vi "check out and in tracking spot.vi"(0 "N spot tracker in":T1, 1 "set state?":bool, 5 "tracking state in":T2={"x state"={"pos estimate"=0.0, "v estimate"=0.0, "weighted position error sum"=0.0, "photon count"=0, "transmit tick count"=0, "axis number"=0, "px (levels^2)"=0.0, "pxv (levels^2/ticks)"=0.0, "pv (levels^2/ticks^2)"=0.0, "vel diff (levels^2/ticks^3)"=0.0, "gx"=0.0, "rtwiddle"=0.0, "photon count ch0"=0, "photon count ch1"=0, "Dx - for pos only k-f"=0.0}, "y state"={"pos estimate"=0.0, "v estimate"=0.0, "weighted position error sum"=0.0, "photon count"=0, "transmit tick count"=0, "axis number"=1, "px (levels^2)"=0.0, "pxv (levels^2/ticks)"=0.0, "pv (levels^2/ticks^2)"=0.0, "vel diff (levels^2/ticks^3)"=0.0, "gx"=0.0, "rtwiddle"=0.0, "photon count ch0"=0, "photon count ch1"=0, "Dx - for pos only k-f"=0.0}, "z state"={"pos estimate"=0.0, "v estimate"=0.0, "weighted position error sum"=0.0, "photon count"=0, "transmit tick count"=0, "axis number"=2, "px (levels^2)"=0.0, "pxv (levels^2/ticks)"=0.0, "pv (levels^2/ticks^2)"=0.0, "vel diff (levels^2/ticks^3)"=0.0, "gx"=0.0, "rtwiddle"=0.0, "photon count ch0"=0, "photon count ch1"=0, "Dx - for pos only k-f"=0.0}}, 7 "new circle":bool, 9 "permission to swap states":bool, 11 "set state value":T2={"x state"={"pos estimate"=0.0, "v estimate"=0.0, "weighted position error sum"=0.0, "photon count"=0, "transmit tick count"=0, "axis number"=0, "px (levels^2)"=0.0, "pxv (levels^2/ticks)"=0.0, "pv (levels^2/ticks^2)"=0.0, "vel diff (levels^2/ticks^3)"=0.0, "gx"=0.0, "rtwiddle"=0.0, "photon count ch0"=0, "photon count ch1"=0, "Dx - for pos only k-f"=0.0}, "y state"={"pos estimate"=0.0, "v estimate"=0.0, "weighted position error sum"=0.0, "photon count"=0, "transmit tick count"=0, "axis number"=1, "px (levels^2)"=0.0, "pxv (levels^2/ticks)"=0.0, "pv (levels^2/ticks^2)"=0.0, "vel diff (levels^2/ticks^3)"=0.0, "gx"=0.0, "rtwiddle"=0.0, "photon count ch0"=0, "photon count ch1"=0, "Dx - for pos only k-f"=0.0}, "z state"={"pos estimate"=0.0, "v estimate"=0.0, "weighted position error sum"=0.0, "photon count"=0, "transmit tick count"=0, "axis number"=2, "px (levels^2)"=0.0, "pxv (levels^2/ticks)"=0.0, "pv (levels^2/ticks^2)"=0.0, "vel diff (levels^2/ticks^3)"=0.0, "gx"=0.0, "rtwiddle"=0.0, "photon count ch0"=0, "photon count ch1"=0, "Dx - for pos only k-f"=0.0}}, 12 "state number to set":u8) -> (4 "N spot tracker out":T1, 6 "tracking state out":T2={"x state"={"pos estimate"=0.0, "v estimate"=0.0, "weighted position error sum"=0.0, "photon count"=0, "transmit tick count"=0, "axis number"=0, "px (levels^2)"=0.0, "pxv (levels^2/ticks)"=0.0, "pv (levels^2/ticks^2)"=0.0, "vel diff (levels^2/ticks^3)"=0.0, "gx"=0.0, "rtwiddle"=0.0, "photon count ch0"=0, "photon count ch1"=0, "Dx - for pos only k-f"=0.0}, "y state"={"pos estimate"=0.0, "v estimate"=0.0, "weighted position error sum"=0.0, "photon count"=0, "transmit tick count"=0, "axis number"=1, "px (levels^2)"=0.0, "pxv (levels^2/ticks)"=0.0, "pv (levels^2/ticks^2)"=0.0, "vel diff (levels^2/ticks^3)"=0.0, "gx"=0.0, "rtwiddle"=0.0, "photon count ch0"=0, "photon count ch1"=0, "Dx - for pos only k-f"=0.0}, "z state"={"pos estimate"=0.0, "v estimate"=0.0, "weighted position error sum"=0.0, "photon count"=0, "transmit tick count"=0, "axis number"=2, "px (levels^2)"=0.0, "pxv (levels^2/ticks)"=0.0, "pv (levels^2/ticks^2)"=0.0, "vel diff (levels^2/ticks^3)"=0.0, "gx"=0.0, "rtwiddle"=0.0, "photon count ch0"=0, "photon count ch1"=0, "Dx - for pos only k-f"=0.0}}, 8 "checked out state number":u8, 10 "use photons to track":bool)   [LabVIEW 2010]
uses:
  kalman 3-axis state.ctl
  integrating single axis kalman state.ctl
  kalman N spot state.ctl
panel:
  in  "tracking?":bool=TRUE
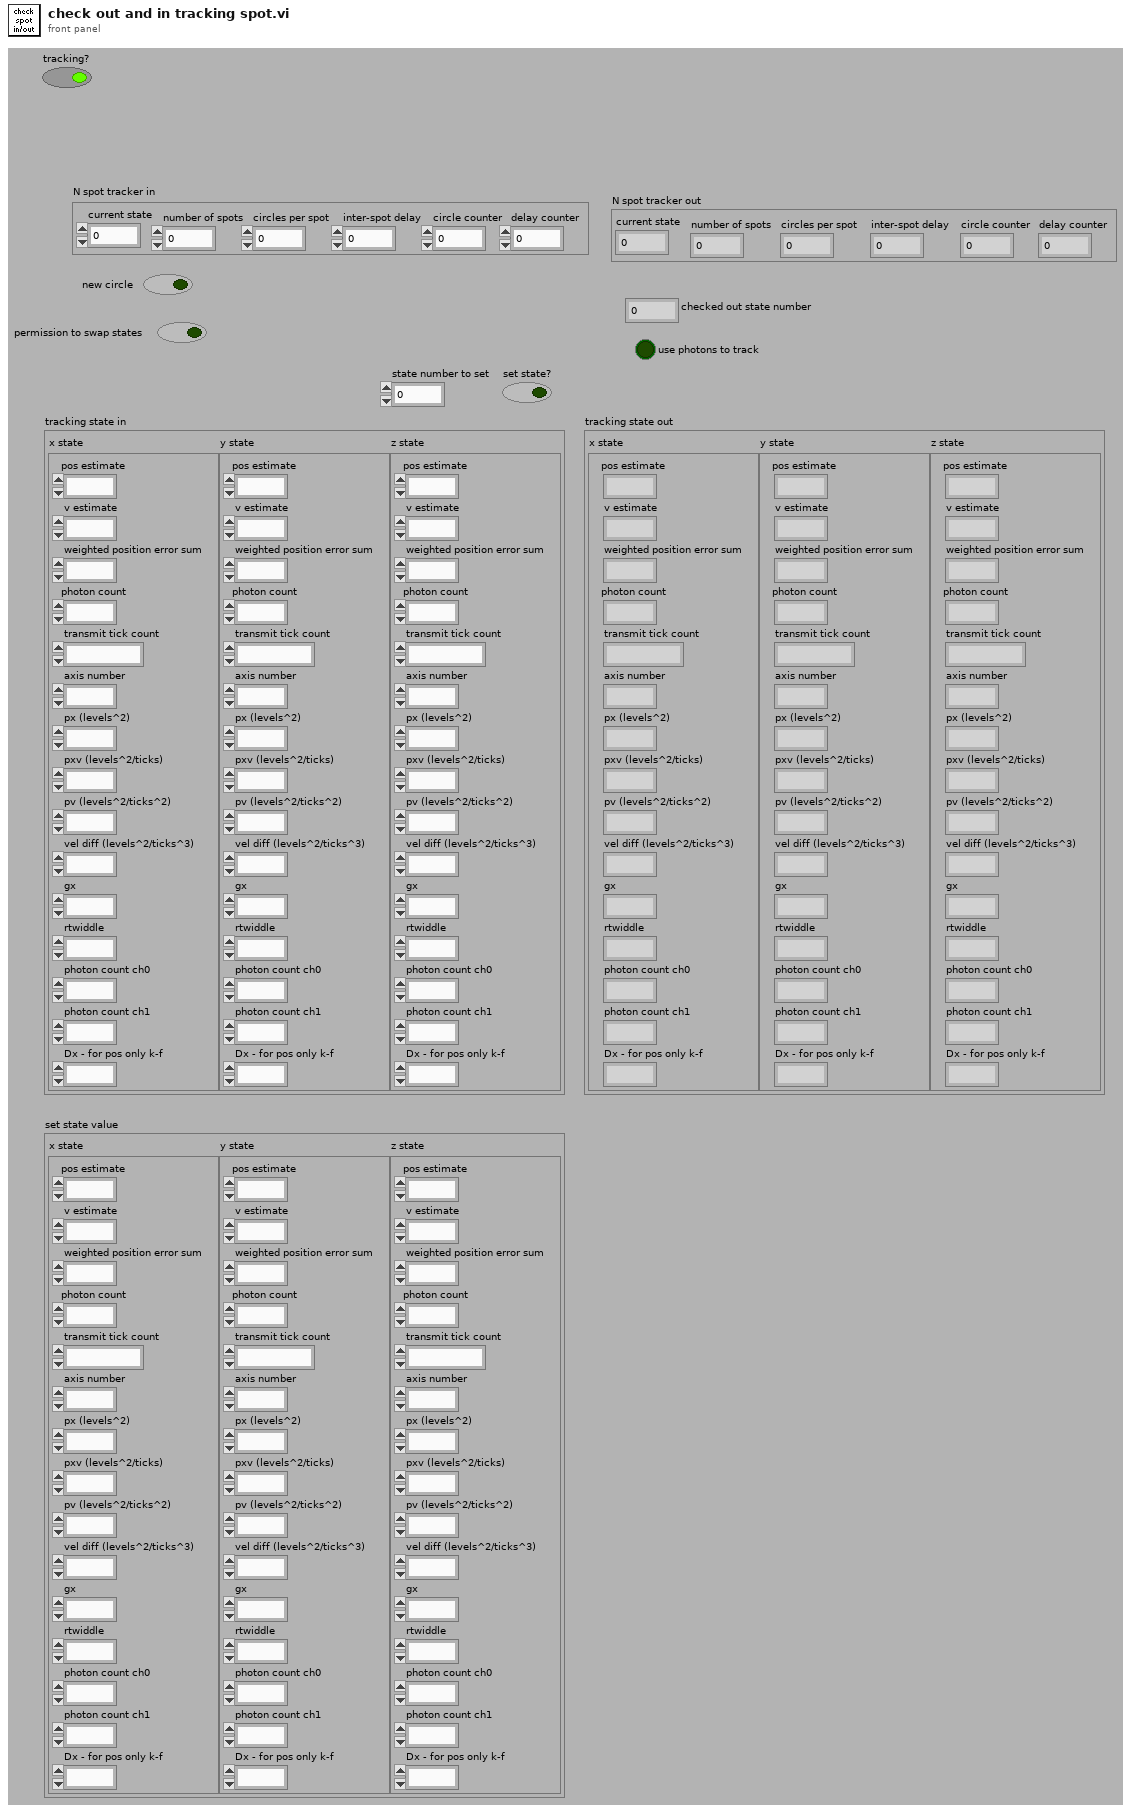
[diagram p1: front panel]
types:
  T1 = typedef "kalman N spot state.ctl" = cluster{"current state":u8, "number of spots":u8, "circles per spot":u8, "inter-spot delay":u8, "circle counter":u8, "delay counter":u8}
  T2 = typedef "kalman 3-axis state.ctl" = cluster{"x state":T3, "y state":T3, "z state":T3}
  T3 = typedef "integrating single axis kalman state.ctl" = cluster{"pos estimate":fxp<+/-,32,16>, "v estimate":fxp<+/-,16,0>, "weighted position error sum":fxp<+/-,32,32>, "photon count":u32, "transmit tick count":u32, "axis number":u8, "px (levels^2)":fxp<+,32,19>, "pxv (levels^2/ticks)":fxp<+,32,2>, "pv (levels^2/ticks^2)":fxp<+,32,-14>, "vel diff (levels^2/ticks^3)":fxp<+,24,-22>, "gx":fxp<+,16,8>, "rtwiddle":fxp<+,16,26>, "photon count ch0":u32, "photon count ch1":u32, "Dx - for pos only k-f":fxp<+,32,19>}
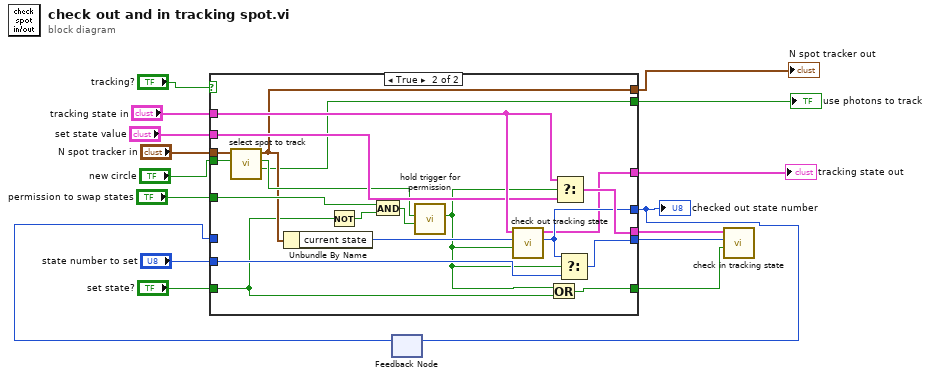
[diagram p0: block diagram]
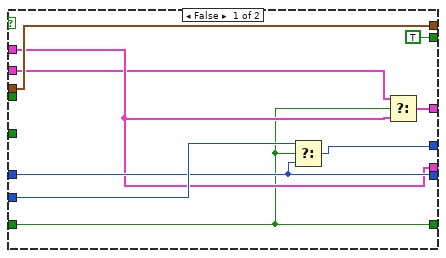
[diagram p2: hidden frame]
diagram:
  n1 = feedback #1() -> (w1:u8)  [unwired: 1 in]
  n2 = case shown="True" "tracking?" {
    tunnel: "tracking state in" -> [w20 w44]
    tunnel: "set state value" -> [w19 w43]
    tunnel: "state number to set" -> [w23 w42]
    tunnel: [w22 w41] -> w13
    tunnel: [w20 w40] -> w12
    tunnel: [w21 w39] -> w2
    tunnel: [w17 w38] -> w11
    tunnel: "N spot tracker in" -> [w25 w37]
    tunnel: "set state?" -> [w18 w27]
    tunnel: "permission to swap states" -> [_ w36]
    tunnel: [w18 w26] -> w3
    tunnel: [w25 w32] -> w7
    tunnel: [TRUE ("use photons to track") w30] -> w6
    tunnel: "new circle" -> [_ w29]
    tunnel: w1 -> [w22 _]
    frame False {
      n3 = Select(t=w23, s=w18, f=w22) -> (s? t:f=w21:u8)
      n4 = Select(t=w19, s=w18, f=w20) -> (s? t:f=w17:T2)
    }
    frame True {
      n5 = call "select spot to track.vi"("new circle"=w29, "N spot tracker in"=w37) -> ("use photons to track"=w30:bool, "state transition"=w33:bool, "N spot tracker out"=w32:T1)  [unwired: 7 in]
      n6 = Unbundle By Name(w32) -> ("current state"=w31:u8)
      n7 = Not(x=w27) -> (.not. x?=w35:bool)
      n8 = And(x=w36, y=w35) -> (x .and. y?=w34:bool)
      n9 = call "hold trigger for permission.vi"("permission"=w34, "trigger"=w33) -> ("trigger out"=w28:bool)  [unwired: 9 in]
      n10 = call "check out tracking state.vi"("check out state"=w28, "state number"=w31, "previous state"=w44) -> ("checked out state number"=w39:u8, "state out"=w38:T2)  [unwired: 7 in]
      n11 = Or(x=w28, y=w27) -> (x .or. y?=w26:bool)
      n12 = Select(t=w44, s=w28, f=w43) -> (s? t:f=w40:T2)
      n13 = Select(t=w39, s=w28, f=w42) -> (s? t:f=w41:u8)
    }
  }
  "tracking state out" <- w11
  "checked out state number" <- w2
  "N spot tracker out" <- w7
  "use photons to track" <- w6
  n14 = feedback-in #1(w2) -> ()
  n15 = call "check in tracking state.vi"("check in state"=w3, "state number"=w13, "state to check in"=w12) -> ()  [unwired: 9 in]
